vi "wheelVelToGlobal.vi"(0 "Utilities in":refnum<class "Utilities.lvclass">, 1 "r_wheel":dbl=1.0 format="%#_13g", 2 "r_robot":dbl=1.0 format="%#_13g", 5 "RobotsFeedback":refnum<class "RobotFeedback.lvclass">[](array[class]), 7 "robotAngles":dbl[](array[numeric])=[30.0, 150.0, 225.0, 315.0] format="%#_13g", 11 "error in (no error)":errorcluster) -> (4 "Utilities out":refnum<class "Utilities.lvclass">, 6 "A x Vector":dbl[][](array[numeric]), 15 "error out":errorcluster)   [LabVIEW 2021, in "Utilities.lvclass"]
uses:
  Utilities.lvclass
  RobotFeedback/RobotFeedback.lvclass
  <vilib>/Analysis/_algsub.llb/Real PseudoInverse Matrix.vi
  <vilib>/Analysis/baseanly.llb/A x Vector.vi
  <vilib>/Analysis/NI_AALPro.lvlib
  <vilib>/Analysis/NI_AALBase.lvlib
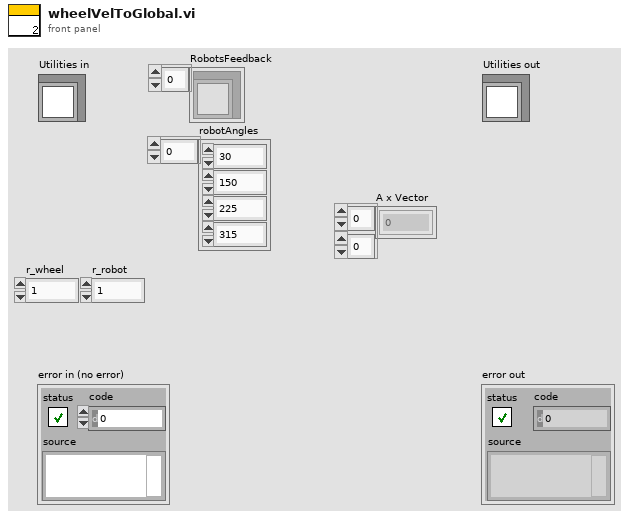
[diagram p1: front panel]
types:
  T1 = typedef "NI_Matrix.lvlib/RealMatrix.ctl" = dbl[][]
  T2 = typedef "feedbackData.ctl" = cluster{"id":u32, "status":u32, "battery":sgl, "encoder1":sgl, "encoder2":sgl, "encoder3":sgl, "encoder4":sgl}
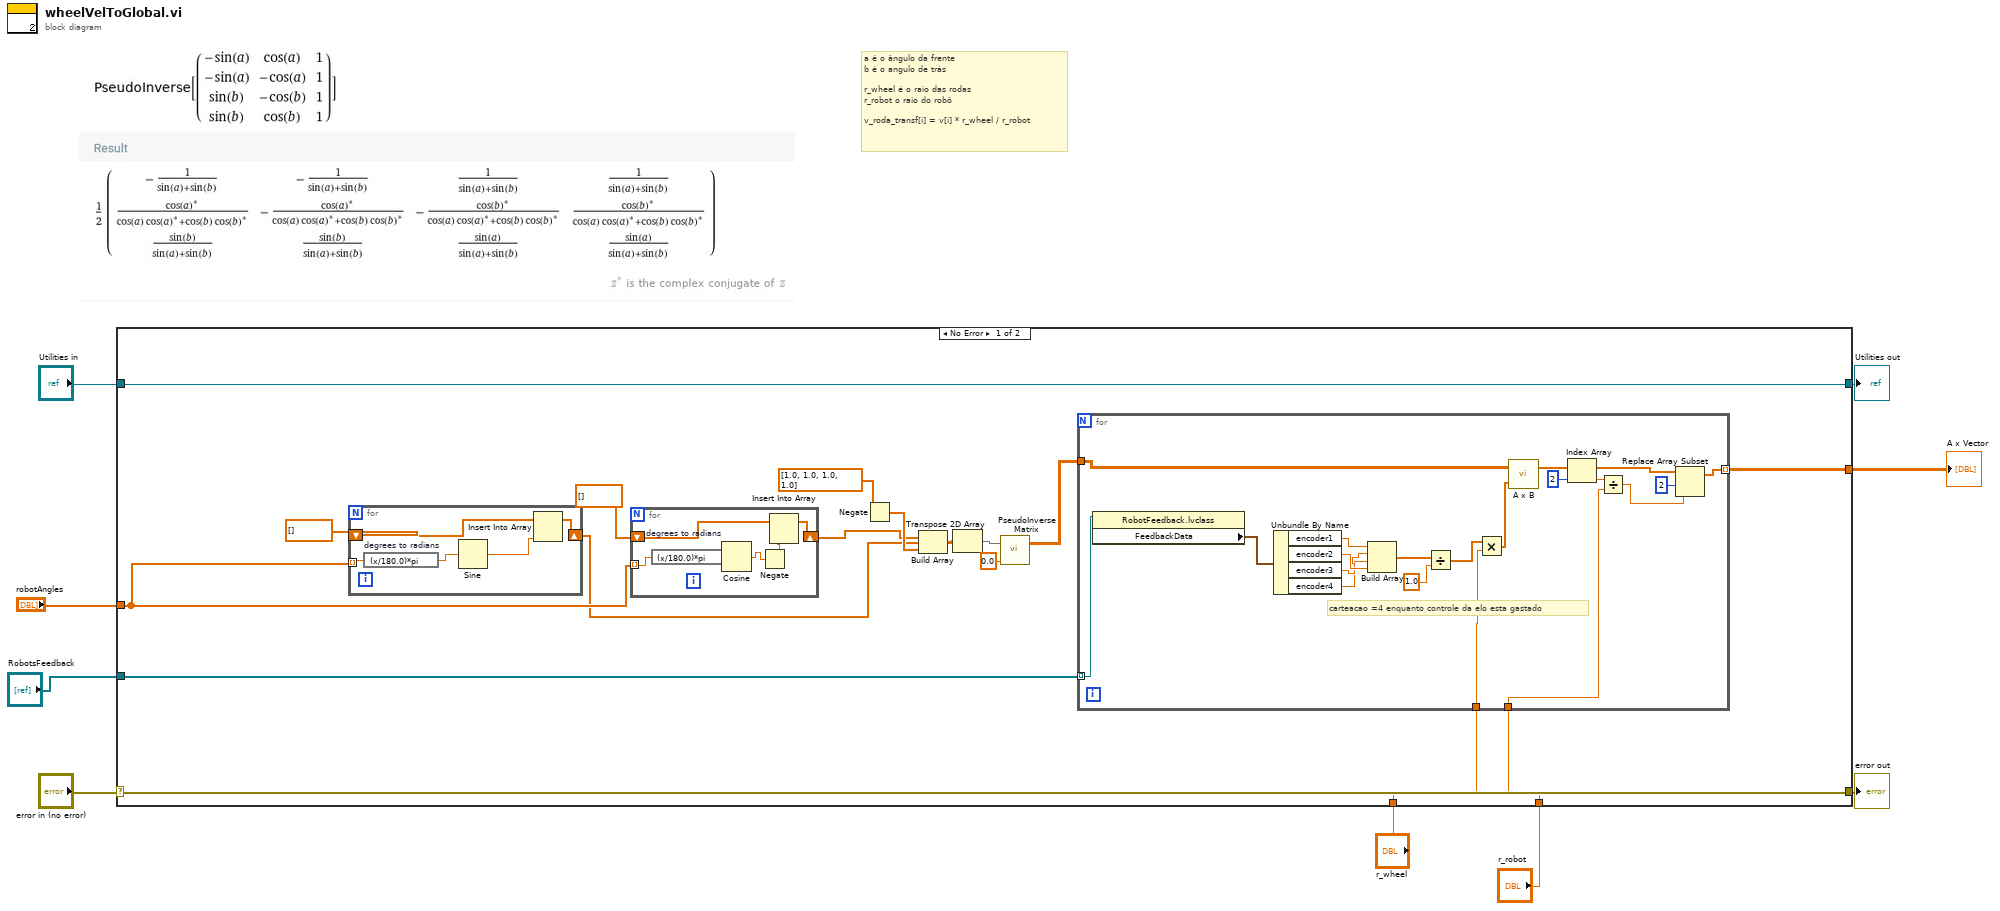
[diagram p0: block diagram]
diagram:
  # "a é o ângulo da frente \nb é o angulo de trás\n\nr_wheel é o raio das rodas\nr_robot o raio do robô\n\nv_roda_transf[i] = v[i] * r_wheel / r_robot"
  n1 = case shown="No Error" "error in (no error)" {
    selector: "error in (no error)" -> [w25 w58]
    tunnel: [w25 w58] -> w8
    tunnel: [w26 w57] -> w6
    tunnel: "Utilities in" -> [w26 w57]
    tunnel: [w18 _] -> w5
    tunnel: "r_robot" -> [w17 _]
    tunnel: "r_wheel" -> [w16 _]
    tunnel: "RobotsFeedback" -> [w15 _]
    tunnel: "robotAngles" -> [w14 _]
    frame No Error {
      n2 = for {
        shift-right: [w55] -> w10
        shift-left: dbl[] [] -> [w56]
        tunnel: w14 -> [w54] mode=indexing
        n3 = expression code="(x/180.0)*pi" "degrees to radians"(w54) -> (w53:dbl)
        n4 = Sine(x=w53) -> (sin(x)=w52:dbl)
        n5 = Insert Into Array(array=w56, new element=w52) -> (w55:dbl[])  [unwired: 1 in]
      }
      n6 = for {
        shift-right: [w50] -> w11
        shift-left: dbl[] [] -> [w51]
        tunnel: w14 -> [w49] mode=indexing
        n7 = expression code="(x/180.0)*pi" "degrees to radians"(w49) -> (w48:dbl)
        n8 = Cosine(x=w48) -> (cos(x)=w47:dbl)
        n9 = Negate(x=w47) -> (-x=w46:dbl)
        n10 = Insert Into Array(array=w51, new element=w46) -> (w50:dbl[])  [unwired: 1 in]
      }
      n11 = Negate(x=dbl[] [1.0, 1.0, 1.0, 1.0] ("Numeric")) -> (-x=w12:dbl[])
      n12 = Build Array(w11, w10, w12) -> (w21:dbl[][])
      n13 = Transpose 2D Array(2D array=w21) -> (transposed array=w20:dbl[][])
      n14 = call-poly <vilib>:"PseudoInverse Matrix.vi"("tolerance"=0.0, "Input Matrix"=w20) -> ("PseudoInverse Matrix"=w19:T1)  [unwired: 1 out]
      n15 = for {
        tunnel: w15 -> [w45] mode=indexing
        tunnel: w19 -> [w43]
        tunnel: [w33] -> w18 mode=indexing
        tunnel: w16 -> [w41]
        tunnel: w17 -> [w35]
        # "carteacao =4 enquanto controle da elo esta gastado"
        n16 = property class="RobotFeedback.lvclass"(reference=w45) -> ("FeedbackData"=w42:T2)  [unwired: 1 in, 2 out]
        n17 = Unbundle By Name(w42) -> ("encoder1"=w44:sgl, "encoder2"=w32:sgl, "encoder3"=w31:sgl, "encoder4"=w30:sgl)
        n18 = Build Array(w44, w31, w30, w32) -> (w29:sgl[])
        n19 = Divide(x=w29, y=1.0) -> (x/y=w27:dbl[])
        n20 = Multiply(x=w27, y=w41) -> (x*y=w40:dbl[])
        n21 = call-poly <vilib>:"A x B.vi"("Vector"=w40, "A"=w43) -> ("A x Vector"=w38:dbl[])  [unwired: 1 out]
        n22 = Index Array(array=w38, index=2) -> (element=w36:dbl)
        n23 = Divide(x=w36, y=w35) -> (x/y=w34:dbl)
        n24 = Replace Array Subset(array=w38, new element=w34, index=2) -> (w33:dbl[])
      }
    }
    frame Error {
    }
  }
  "error out" <- w8
  "Utilities out" <- w6
  "A x Vector" <- w5
